vi "Global_1.vi"() -> ()   [LabVIEW 2019]
panel:
  in  "Prev Boolean":bool
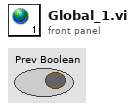
[diagram p1: front panel]
diagram:
